vi "ArduinoRead.vi"(7 "Arduino function":enum16{"T/RH", "Interlock", "Edgesense"}(ring), 8 "error in (no error)":errorcluster, 9 "Humidity IN":dbl[](array[numeric]), 10 "Temperature IN":dbl[](array[numeric]), 11 "ArduinoControl in":refnum<class "ArduinoControl.lvclass">) -> (0 "error out":errorcluster, 1 "rel. Humidity [%]":dbl, 2 "Temperature [°C]":dbl, 3 "ArduinoControl out":refnum<class "ArduinoControl.lvclass">, 4 "Interlock Status":u16(ring) items=["Dark", "Light"], 5 "Edgesense Status":u16(ring)=1 items=["Contact", "No contact"])   [LabVIEW 2013, in "ArduinoControl.lvclass"]
uses:
  ArduinoControl.lvclass
  ArduinoControl.lvclass/ArduinoControl.ctl
panel:
  out "Humidity OUT":dbl[](array[numeric])
  out "Temperature OUT":dbl[](array[numeric])
  out "return count":u32
  out "String":string
  out "VISA resource name OUT":refnum<visa-resource-name>="COM24"
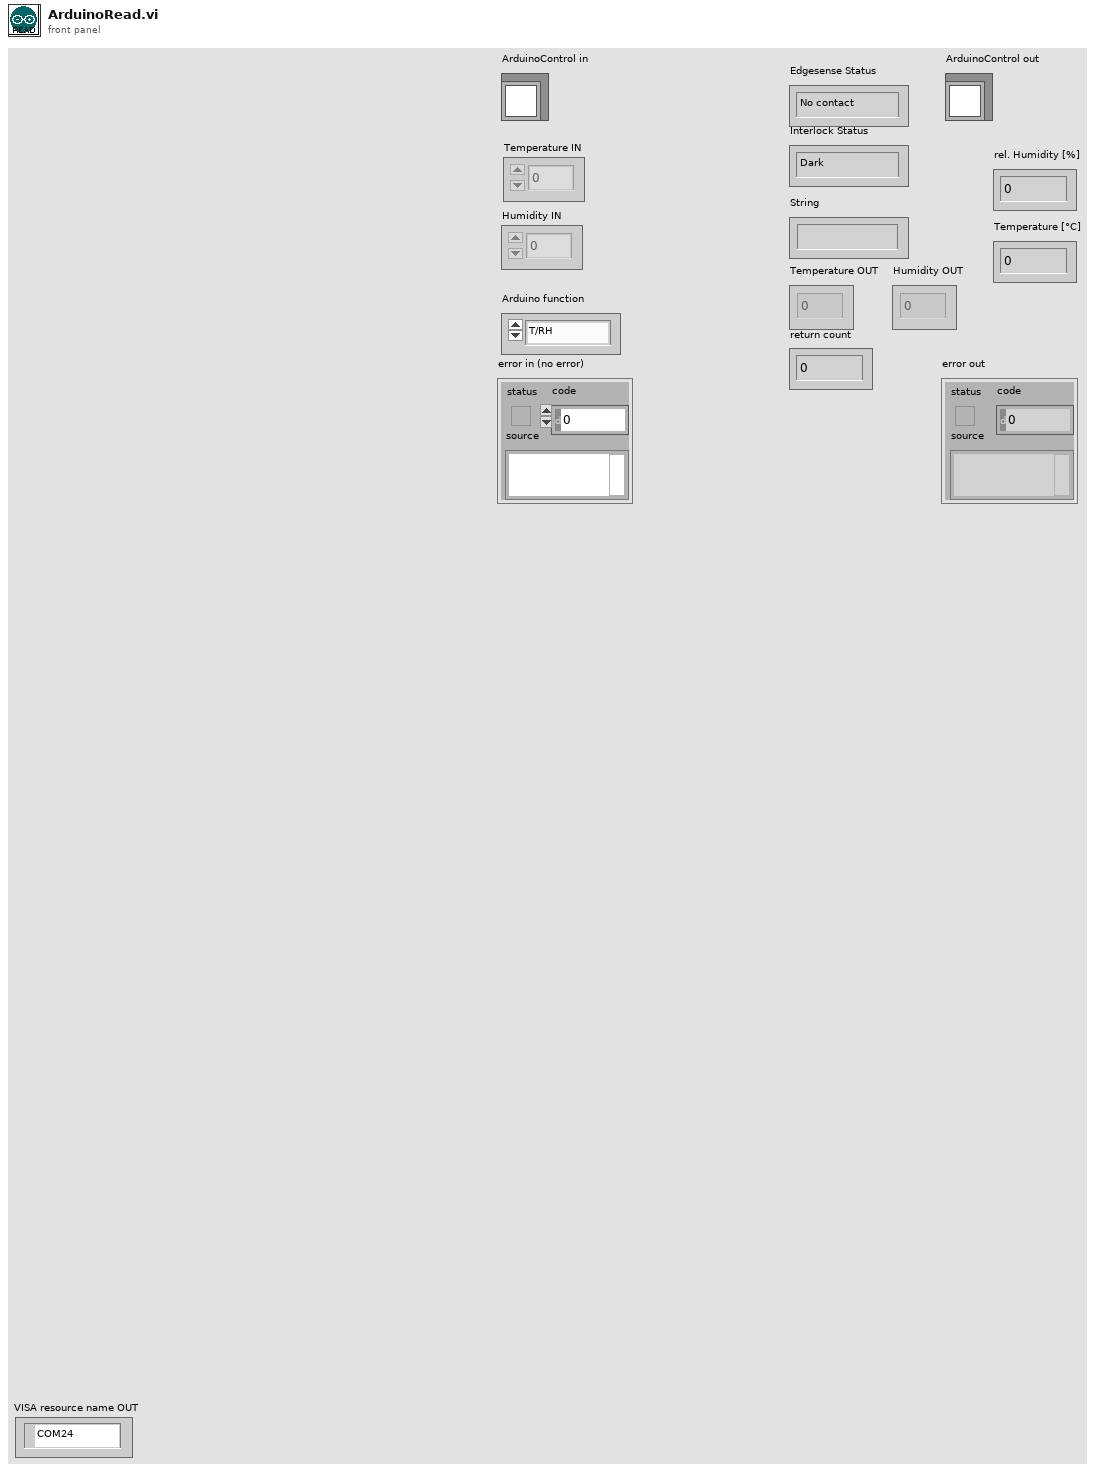
[diagram p1: front panel]
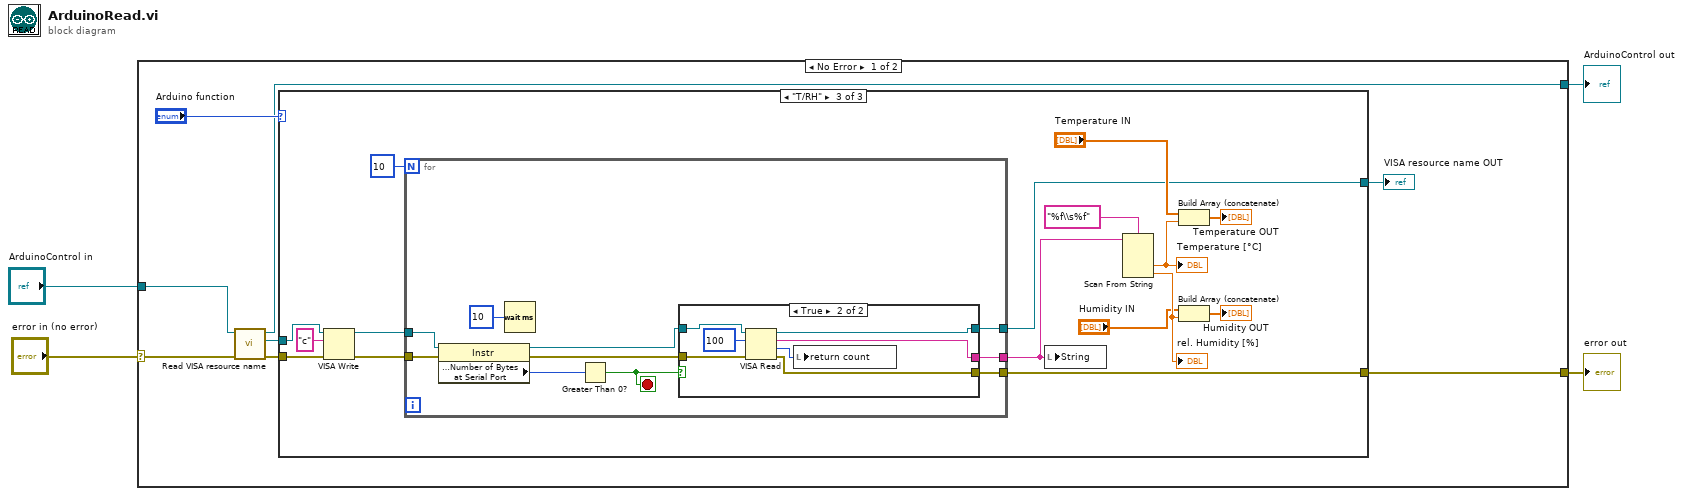
[diagram p0: block diagram]
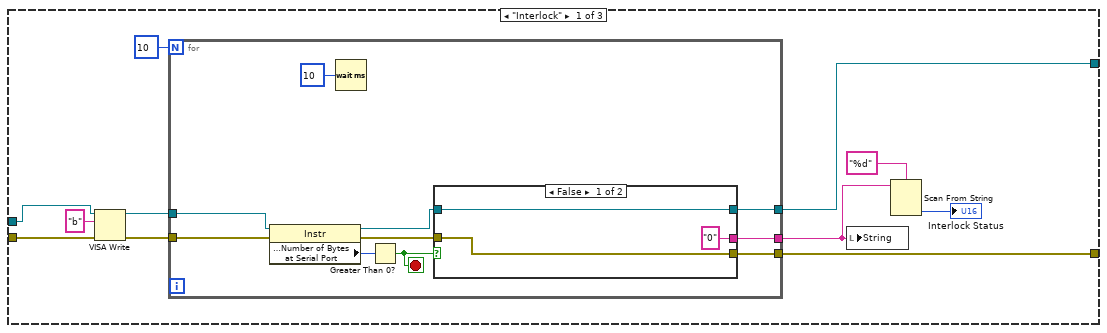
[diagram p2: hidden frame]
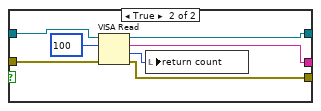
[diagram p3: hidden frame]
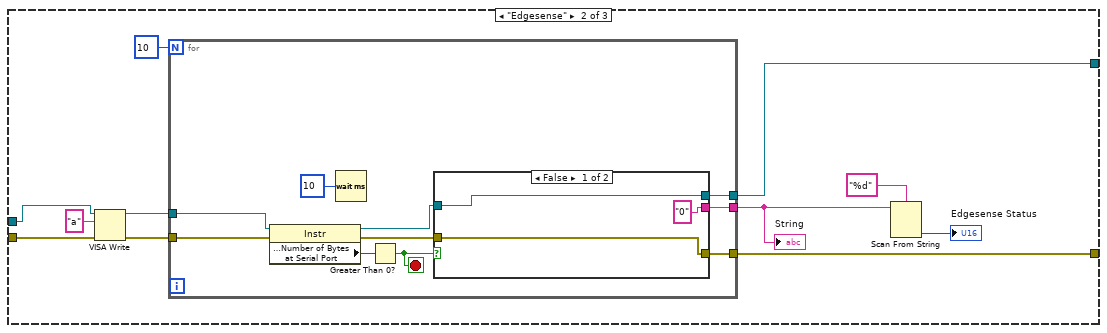
[diagram p4: hidden frame]
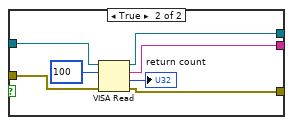
[diagram p5: hidden frame]
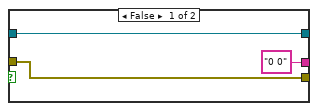
[diagram p6: hidden frame]
diagram:
  n1 = case shown="No Error" "error in (no error)" {
    selector: "error in (no error)" -> [w7 w112]
    tunnel: [w8 w111] -> w2
    tunnel: "ArduinoControl in" -> [w9 w111]
    tunnel: [w10 w112] -> w1
    frame No Error {
      n2 = call "Read VISA resource name.vi"("error in (no error)"=w7, "ArduinoControl in"=w9) -> ("error out"=w6:errorcluster, "VISA resource name"=w5:refnum<visa-resource-name>, "ArduinoControl out"=w8:refnum<class "ArduinoControl.lvclass">)  [unwired: 7 in]
      n3 = case shown="\"T/RH\"" "Arduino function" {
        tunnel: w6 -> [w15 w47 w78]
        tunnel: w5 -> [w17 w48 w80]
        tunnel: [w20 w50 w81] -> w11
        tunnel: [w19 w51 w82] -> w10
        frame "Interlock" {
          n4 = VISA Write(VISA resource name=w17, write buffer="b", error in (no error)=w15) -> (VISA resource name out=w16:refnum<visa-resource-name>, error out=w14:errorcluster)  [unwired: 1 out]
          n5 = for {
            N: 10 -> [_]
            tunnel: [w31] -> w20
            tunnel: [w30] -> w21
            tunnel: w14 -> [w25]
            tunnel: w16 -> [w26]
            tunnel: [w29] -> w19
            stop <- w24 stop-if-true
            n6 = property class="Instr"(reference=w26, error in=w25) -> (reference out=w33:refnum<visa-resource-name>, error out=w32:errorcluster, "Serial Settings:Number of Bytes at Serial Port"=w27:u32)
            n7 = Wait (ms)(milliseconds to wait=10) -> ()  [unwired: 1 out]
            n8 = Greater Than 0?(x=w27) -> (x > 0?=w24:bool)
            n9 = case shown="False" w24 {
              tunnel: w33 -> [w35 w43]
              tunnel: w32 -> [w36 w42]
              tunnel: [w35 w41] -> w31
              tunnel: ["0" w40] -> w30
              tunnel: [w36 w39] -> w29
              frame False {
              }
              frame True {
                n10 = VISA Read(VISA resource name=w43, byte count=100, error in (no error)=w42) -> (VISA resource name out=w41:refnum<visa-resource-name>, read buffer=w40:string, return count=w38:u32, error out=w39:errorcluster)
                n11 = local write "return count"(w38) -> ()
              }
            }
          }
          n12 = local write "String"(w21) -> ()
          n13 = Scan From String(format string="%d", input string=w21) -> (output 1=→"Interlock Status":u16)  [unwired: 3 in, 3 out]
        }
        frame "Edgesense" {
          n14 = VISA Write(VISA resource name=w48, write buffer="a", error in (no error)=w47) -> (VISA resource name out=w46:refnum<visa-resource-name>, error out=w45:errorcluster)  [unwired: 1 out]
          n15 = for {
            N: 10 -> [_]
            tunnel: [w62] -> w50
            tunnel: [w61] -> w52
            tunnel: w46 -> [w57]
            tunnel: [w60] -> w51
            tunnel: w45 -> [w58]
            stop <- w55 stop-if-true
            n16 = property class="Instr"(reference=w57, error in=w58) -> (reference out=w64:refnum<visa-resource-name>, error out=w63:errorcluster, "Serial Settings:Number of Bytes at Serial Port"=w56:u32)
            n17 = Wait (ms)(milliseconds to wait=10) -> ()  [unwired: 1 out]
            n18 = Greater Than 0?(x=w56) -> (x > 0?=w55:bool)
            n19 = case shown="False" w55 {
              tunnel: w64 -> [w66 w74]
              tunnel: w63 -> [w67 w73]
              tunnel: [w66 w72] -> w62
              tunnel: ["0" w71] -> w61
              tunnel: [w67 w70] -> w60
              frame False {
              }
              frame True {
                n20 = VISA Read(VISA resource name=w74, byte count=100, error in (no error)=w73) -> (VISA resource name out=w72:refnum<visa-resource-name>, read buffer=w71:string, return count=→"return count":u32, error out=w70:errorcluster)
              }
            }
          }
          "String" <- w52
          n21 = Scan From String(format string="%d", input string=w52) -> (output 1=→"Edgesense Status":u16)  [unwired: 3 in, 3 out]
        }
        frame "T/RH" {
          n22 = VISA Write(VISA resource name=w80, write buffer="c", error in (no error)=w78) -> (VISA resource name out=w76:refnum<visa-resource-name>, error out=w77:errorcluster)  [unwired: 1 out]
          n23 = for {
            N: 10 -> [_]
            tunnel: [w98] -> w81
            tunnel: [w97] -> w83
            tunnel: w77 -> [w93]
            tunnel: w76 -> [w92]
            tunnel: [w96] -> w82
            stop <- w91 stop-if-true
            n24 = property class="Instr"(reference=w92, error in=w93) -> (reference out=w100:refnum<visa-resource-name>, error out=w99:errorcluster, "Serial Settings:Number of Bytes at Serial Port"=w94:u32)
            n25 = Wait (ms)(milliseconds to wait=10) -> ()  [unwired: 1 out]
            n26 = Greater Than 0?(x=w94) -> (x > 0?=w91:bool)
            n27 = case shown="True" w91 {
              tunnel: w100 -> [w102 w110]
              tunnel: w99 -> [w103 w109]
              tunnel: [w102 w108] -> w98
              tunnel: ["0 0" w107] -> w97
              tunnel: [w103 w106] -> w96
              frame False {
              }
              frame True {
                n28 = VISA Read(VISA resource name=w110, byte count=100, error in (no error)=w109) -> (VISA resource name out=w108:refnum<visa-resource-name>, read buffer=w107:string, return count=w104:u32, error out=w106:errorcluster)
                n29 = local write "return count"(w104) -> ()
              }
            }
          }
          n30 = local write "String"(w83) -> ()
          n31 = Scan From String(format string="%f\\s%f", input string=w83) -> (output 1=w85:dbl, output 2=w90:dbl)  [unwired: 4 in, 3 out]
          "rel. Humidity [%]" <- w90
          "Temperature [°C]" <- w85
          n32 = Build Array (concatenate)("Temperature IN", w85) -> (→"Temperature OUT":dbl[])
          n33 = Build Array (concatenate)("Humidity IN", w90) -> (→"Humidity OUT":dbl[])
        }
      }
      "VISA resource name OUT" <- w11
    }
    frame Error {
    }
  }
  "error out" <- w1
  "ArduinoControl out" <- w2
